vi "get waveform - 8bit.vi"(8 "error in (no error)":errorcluster caption="에러 입력(에러 없음)", 11 "PWL_DW7802 입력":refnum<class "PWL_DW7802.lvclass">) -> (0 "error out":errorcluster caption="에러 출력", 1 "8bit memory data":u8[](array[numeric]), 2 "8bit waveform":waveform(i8), 3 "PWL_DW7802 출력":refnum<class "PWL_DW7802.lvclass">)   [LabVIEW 2020, in "PWL_DW7802.lvclass"]
uses:
  PWL_DW7802.lvclass
  Waveform Gen/Waveform Gen.lvclass/Waveform Gen.ctl
  PWL/PWL.lvclass/PWL.ctl
  Waveform Gen/Accessors/Read scale.vi
  PWL/Accessors/Read waveform type.vi
  Waveform Gen/Accessors/Read repeat type.vi
  Waveform Gen/Accessors/Read frequency.vi
  Waveform Gen/Accessors/Read cycle.vi
  PWL/PWL.lvclass
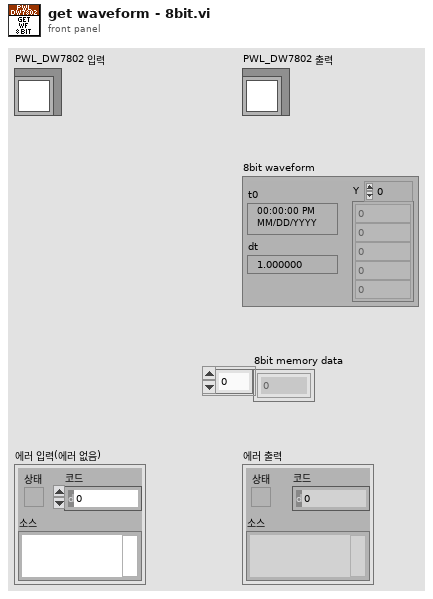
[diagram p1: front panel]
types:
  T1 = typedef "Waveform Gen.lvclass/waveform gen type.ctl" = enum16{"Sine", "Square", "Triangle", "Sawtooth", "Auto Track", "Auto Brake (Square)", "Auto Brake (Sine)", "PWL"}
  T2 = typedef "Waveform Gen.lvclass/repeat scale.ctl" = enum16{"Normal", "Lin. Up", "Lin. Down", "Exp. Up", "Exp. Down"}
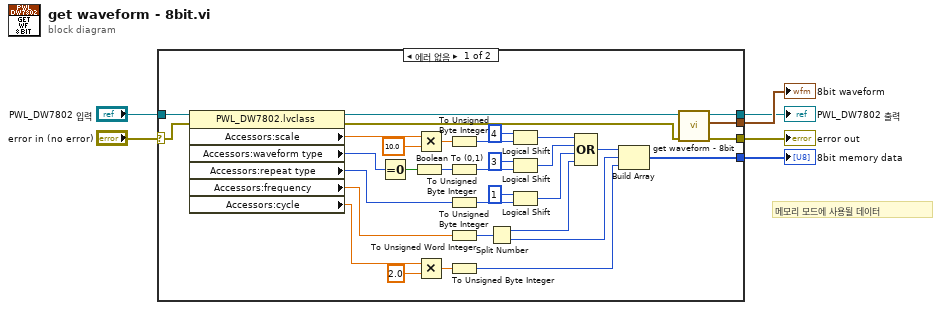
[diagram p0: block diagram]
diagram:
  # "메모리 모드에 사용될 데이터"
  n1 = case shown="에러 없음" "error in (no error)" {
    selector: "error in (no error)" -> [w34 w40]
    tunnel: [w39 w40] -> w6
    tunnel: [w38 _] -> w5
    tunnel: [w37 w41] -> w4
    tunnel: "PWL_DW7802 입력" -> [w36 w41]
    tunnel: [w11 _] -> w1
    frame No Error {
      n2 = property class="PWL_DW7802.lvclass"(reference=w36, error in=w34) -> (reference out=w35:refnum<class "PWL_DW7802.lvclass">, error out=w33:errorcluster, "Accessors:scale"=w32:dbl, "Accessors:waveform type"=w29:T1, "Accessors:repeat type"=w26:T2, "Accessors:frequency"=w28:dbl, "Accessors:cycle"=w27:dbl)
      n3 = Equal To 0?(x=w29) -> (x = 0?=w8:bool)
      n4 = Boolean To (0,1)(Boolean=w8) -> (0, 1=w7:i16)
      n5 = Multiply(x=w32, y=10.0) -> (x*y=w30:dbl)
      n6 = Multiply(x=w27, y=2.0) -> (x*y=w10:dbl)
      n7 = To Unsigned Byte Integer(number=w30) -> (unsigned 8bit integer=w20:u8)
      n8 = To Unsigned Byte Integer(number=w7) -> (unsigned 8bit integer=w18:u8)
      n9 = To Unsigned Byte Integer(number=w26) -> (unsigned 8bit integer=w16:u8)
      n10 = To Unsigned Word Integer(number=w28) -> (unsigned 16bit integer=w25:u16)
      n11 = To Unsigned Byte Integer(number=w10) -> (unsigned 8bit integer=w21:u8)
      n12 = Split Number(x=w25) -> (hi(x)=w24:u8, lo(x)=w22:u8)
      n13 = Logical Shift(y=i16 4, x=w20) -> (x << y=w12:u8)
      n14 = Logical Shift(y=i16 3, x=w18) -> (x << y=w13:u8)
      n15 = Logical Shift(y=i16 1, x=w16) -> (x << y=w14:u8)
      n16 = Compound Arithmetic op=OR(w12, w13, w14, w24) -> (w23:u8)
      n17 = Build Array(w23, w22, w21) -> (w11:u8[])
      n18 = call-parent "get waveform - 8bit.vi"("error in (no error)"=w33, "Waveform Obj 입력"=w35) -> ("error out"=w39:errorcluster, "8bit waveform"=w38:waveform(i8), "Waveform Obj 출력"=w37:refnum<class "PWL_DW7802.lvclass">)  [unwired: 6 in, 1 out]
    }
    frame Error {
    }
  }
  "error out" <- w6
  "PWL_DW7802 출력" <- w4
  "8bit waveform" <- w5
  "8bit memory data" <- w1
